vi "Slave Master.vi"() -> ()   [LabVIEW 2012]
uses:
  MyGlobals.vi
panel:
  out "Final String":string
  out "Original String":string
  in  "Enter String":string="Hello "
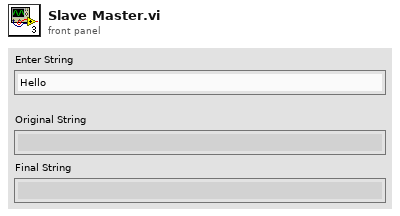
[diagram p1: front panel]
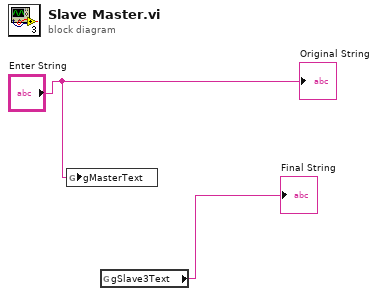
[diagram p0: block diagram]
diagram:
  n1 = global write "MyGlobals.vi" "gMasterText"("Enter String") -> ()
  n2 = global read "MyGlobals.vi" "gSlave3Text"() -> (→"Final String":string)
  "Original String" <- "Enter String"
